vi "teste sequencia.vi"() -> ()   [LabVIEW 2018]
panel:
  in  "stop":bool
  in  "Boolean":bool
  in  "Select Test":T1(ring)
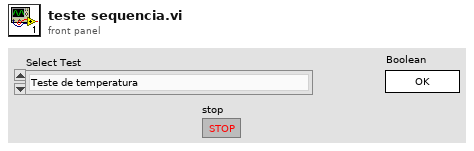
[diagram p1: front panel]
types:
  T1 = enum16{"Teste de temperatura", "Teste de pressão"}
  T2 = enum32{"Invalid", "Standard", "Closed", "Hidden", "Minimized", "Maximized"}
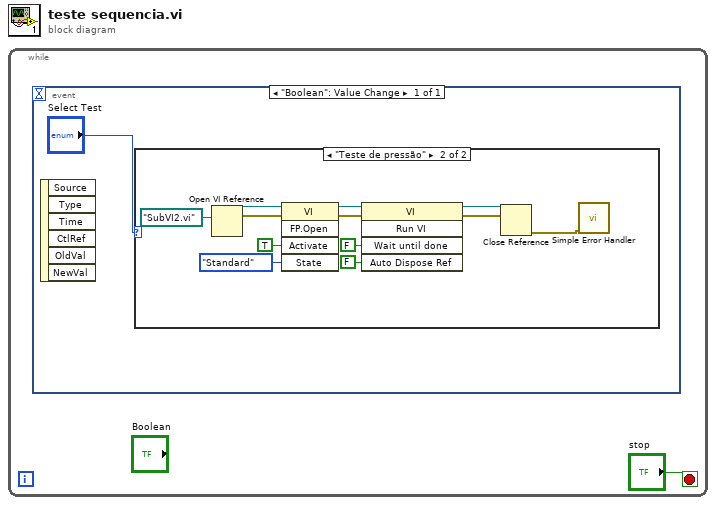
[diagram p0: block diagram]
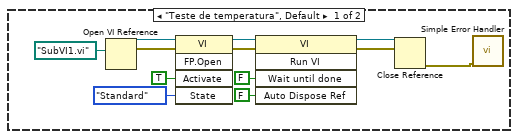
[diagram p2: hidden frame]
diagram:
  n1 = while {
    stop <- "stop" stop-if-true
    n2 = event shown="[0] \"Boolean\": Value Change" {
      selector: _ -> [_]
      dyn-events: _ -> [_]
      timeout: _ -> [_]
      event "Boolean": Value Change {
        n3 = event-data() -> ()  [unwired: 1 in, 6 out]
        n4 = case shown="\"Teste de pressão\"" "Select Test" {
          frame "Teste de temperatura", Default {
            n5 = Open VI Reference(vi path=path "SubVI1.vi") -> (vi reference=w13:refnum<vi>, error out=w12:errorcluster)  [unwired: 5 in]
            n6 = invoke class="VI" method="FP.Open"(reference=w13, error in=w12, "Activate"=TRUE ("Activate?"), "State"=T2."Standard") -> (reference out=w9:refnum<vi>, error out=w8:errorcluster)  [unwired: 1 in, 3 out]
            n7 = invoke class="VI" method="Run VI"(reference=w9, error in=w8, "Wait until done"=FALSE ("Wait Until Done"), "Auto Dispose Ref"=FALSE ("Auto Dispose Reference")) -> (reference out=w5:refnum<vi>, error out=w4:errorcluster)  [unwired: 1 in, 3 out]
            n8 = Close Reference(reference=w5, error in (no error)=w4) -> (error out=w3:errorcluster)
            n9 = call <vilib>:"Simple Error Handler.vi"("error in (no error)"=w3) -> ()  [unwired: 4 in, 5 out]
          }
          frame "Teste de pressão" {
            n10 = Open VI Reference(vi path=path "SubVI2.vi") -> (vi reference=w25:refnum<vi>, error out=w24:errorcluster)  [unwired: 5 in]
            n11 = invoke class="VI" method="FP.Open"(reference=w25, error in=w24, "Activate"=TRUE ("Activate?"), "State"=T2."Standard") -> (reference out=w21:refnum<vi>, error out=w20:errorcluster)  [unwired: 1 in, 3 out]
            n12 = invoke class="VI" method="Run VI"(reference=w21, error in=w20, "Wait until done"=FALSE ("Wait Until Done"), "Auto Dispose Ref"=FALSE ("Auto Dispose Reference")) -> (reference out=w17:refnum<vi>, error out=w16:errorcluster)  [unwired: 1 in, 3 out]
            n13 = Close Reference(reference=w17, error in (no error)=w16) -> (error out=w15:errorcluster)
            n14 = call <vilib>:"Simple Error Handler.vi"("error in (no error)"=w15) -> ()  [unwired: 4 in, 5 out]
          }
        }
      }
    }
  }
